vi "Lab Panel V5.29.vi"() -> ()   [LabVIEW 2013] (continued)
            n2896 = Unbundle(w5232) -> ("OUT SERVER ADDRESS"=w5231:string, "FROM ACCOUNT"=w5230:string, "TEST MAIL"=w5229:bool)  [unwired: 4 out]
            n2897 = stacked-sequence {
              tunnel: "TO (string):" -> [_ w5271]
              tunnel: w5232 -> [w5237 w5270]
              tunnel: w5231 -> [w5236 w5269]
              tunnel: w5230 -> [w5235 w5268]
              tunnel: w5229 -> [w5234 _]
              tunnel: w5218 -> [_ w5267]
              tunnel: w5228 -> [_ w5266]
              tunnel: w5227 -> [_ w5265]
              tunnel: w5226 -> [_ w5264]
              tunnel: w5225 -> [_ w5263]
              tunnel: w5224 -> [_ w5262]
              tunnel: w5223 -> [_ w5261]
              tunnel: w5222 -> [_ w5260]
              tunnel: w5221 -> [_ w5259]
              tunnel: w5220 -> [_ w5258]
              tunnel: w5219 -> [_ w5257]
              tunnel: "TO (string):" -> [w5233 _]
              frame #0 {
                # "mail test"
                n2898 = case shown="True" w5234 {
                  tunnel: w5237 -> [_ w5241]
                  tunnel: w5233 -> [_ w5240]
                  tunnel: w5236 -> [_ w5239]
                  tunnel: w5235 -> [_ w5238]
                  frame False {
                  }
                  frame True {
                    n2899 = stacked-sequence {
                      seq-local: [_ _ w5251 _] -> [_ _ _ w5252]
                      tunnel: w5241 -> [w5244 _ _ w5256]
                      tunnel: w5240 -> [_ _ w5249 _]
                      tunnel: w5239 -> [_ _ w5247 _]
                      tunnel: w5238 -> [_ _ w5248 _]
                      frame #0 {
                        n2900 = Bundle(cluster=w5244, "TEST MAIL STATUS"="TEST START") -> (w5242:T7)  [unwired: 6 in]
                        n2901 = local write "MAIL SETTINGS"(w5242) -> ()
                      }
                      frame #1 {
                        n2902 = Wait (ms)(milliseconds to wait=500) -> ()  [unwired: 1 out]
                      }
                      frame #2 {
                        n2903 = call "sub vi - send mail v5.vi"("TO:"=w5249, "subject"="MAIL TEST FROM LAB PANEL", "from"=w5248, "out going server"=w5247, "message"="TEST MESSAGE") -> ("error out"=w5251:errorcluster)  [unwired: 10 in]
                      }
                      frame #3 {
                        n2904 = Bundle(cluster=w5256, "TEST MAIL"=FALSE, "TEST MAIL STATUS"="TEST END", "mail error"=w5252) -> (w5254:T7)  [unwired: 4 in]
                        n2905 = local write "MAIL SETTINGS"(w5254) -> ()
                      }
                    }
                  }
                }
              }
              frame #1 {
                # "mail report"
                n2906 = stacked-sequence {
                  seq-local: [_ w5314 _ _] -> [_ _ _ w5504]
                  seq-local: [_ _ w5417 _] -> [_ _ _ w5494]
                  seq-local: [w5281 _ _ _] -> [_ w5331 _ _]
                  seq-local: [w5280 _ _ _] -> [_ w5330 _ _]
                  seq-local: [w5278 _ _ _] -> [_ w5328 _ _]
                  seq-local: [w5279 _ _ _] -> [_ w5329 _ _]
                  seq-local: [w5277 _ _ _] -> [_ w5327 _ _]
                  seq-local: [w5276 _ _ _] -> [_ w5322 _ _]
                  seq-local: [w5275 _ _ _] -> [_ w5323 _ _]
                  seq-local: [w5274 _ _ _] -> [_ w5324 _ _]
                  seq-local: [w5273 _ _ _] -> [_ w5325 _ _]
                  seq-local: [w5272 _ _ _] -> [_ w5326 _ _]
                  tunnel: w5271 -> [_ _ _ w5505]
                  tunnel: w5270 -> [_ _ _ w5488]
                  tunnel: w5269 -> [_ _ _ w5502]
                  tunnel: w5268 -> [_ _ _ w5501]
                  tunnel: w5267 -> [w5312 _ _ w5496]
                  tunnel: w5266 -> [_ _ w5447 _]
                  tunnel: w5265 -> [_ _ w5444 _]
                  tunnel: w5264 -> [_ _ w5443 _]
                  tunnel: w5263 -> [_ _ w5442 _]
                  tunnel: w5262 -> [_ _ w5441 _]
                  tunnel: w5261 -> [_ _ w5440 _]
                  tunnel: w5260 -> [_ _ w5439 _]
                  tunnel: w5259 -> [_ _ w5438 _]
                  tunnel: w5258 -> [_ _ w5437 _]
                  tunnel: w5257 -> [_ _ w5436 _]
                  frame #0 {
                    n2907 = case shown="False" w5312 {
                      frame False {
                        n2908 = local write "mail control"("") -> ()
                      }
                      frame True {
                      }
                    }
                    n2909 = local read "SET LAB01-1"() -> (w5311:T5)
                    n2910 = local read "SET LAB01-2"() -> (w5310:T5)
                    n2911 = local read "SET LAB02-1"() -> (w5309:T5)
                    n2912 = local read "SET LAB02-2"() -> (w5308:T5)
                    n2913 = local read "SET LAB03-1"() -> (w5307:T5)
                    n2914 = local read "SET LAB04-1"() -> (w5305:T5)
                    n2915 = local read "SET LAB05-1"() -> (w5303:T5)
                    n2916 = local read "SET LAB03-2"() -> (w5306:T5)
                    n2917 = local read "SET LAB04-2"() -> (w5304:T5)
                    n2918 = local read "SET LAB05-2"() -> (w5302:T5)
                    n2919 = Unbundle(w5307) -> ("DESCRIPTION"=w5287:string)  [unwired: 4 out]
                    n2920 = Unbundle(w5306) -> ("DESCRIPTION"=w5286:string)  [unwired: 4 out]
                    n2921 = Unbundle(w5305) -> ("DESCRIPTION"=w5285:string)  [unwired: 4 out]
                    n2922 = Unbundle(w5302) -> ("DESCRIPTION"=w5282:string)  [unwired: 4 out]
                    n2923 = Unbundle(w5308) -> ("DESCRIPTION"=w5288:string)  [unwired: 4 out]
                    n2924 = Unbundle(w5304) -> ("DESCRIPTION"=w5284:string)  [unwired: 4 out]
                    n2925 = Unbundle(w5311) -> ("DESCRIPTION"=w5300:string)  [unwired: 4 out]
                    n2926 = Unbundle(w5309) -> ("DESCRIPTION"=w5289:string)  [unwired: 4 out]
                    n2927 = Unbundle(w5303) -> ("DESCRIPTION"=w5283:string)  [unwired: 4 out]
                    n2928 = Unbundle(w5310) -> ("DESCRIPTION"=w5290:string)  [unwired: 4 out]
                    n2929 = Concatenate Strings("[LAB05-2/", w5282) -> (w5272:string)
                    n2930 = Concatenate Strings("[LAB05-1/", w5283) -> (w5273:string)
                    n2931 = Concatenate Strings("[LAB04-2/", w5284) -> (w5274:string)
                    n2932 = Concatenate Strings("[LAB03-2/", w5286) -> (w5276:string)
                    n2933 = Concatenate Strings("[LAB04-1/", w5285) -> (w5275:string)
                    n2934 = Concatenate Strings("[LAB03-1/", w5287) -> (w5277:string)
                    n2935 = Concatenate Strings("[LAB01-2/", w5290) -> (w5280:string)
                    n2936 = Concatenate Strings("[LAB02-2/", w5288) -> (w5278:string)
                    n2937 = Concatenate Strings("[LAB01-1/", w5300) -> (w5281:string)
                    n2938 = Concatenate Strings("[LAB02-1/", w5289) -> (w5279:string)
                  }
                  frame #1 {
                    w5335 = "/"
                    w5336 = 2.0
                    n2939 = local read "DISP LAB01-2"() -> (w5415:T4)
                    n2940 = local read "DISP LAB01-1"() -> (w5416:T4)
                    n2941 = local read "DISP LAB02-1"() -> (w5414:T4)
                    n2942 = local read "DISP LAB03-2"() -> (w5411:T4)
                    n2943 = local read "DISP LAB02-2"() -> (w5413:T4)
                    n2944 = local read "DISP LAB03-1"() -> (w5412:T4)
                    n2945 = local read "DISP LAB04-2"() -> (w5409:T4)
                    n2946 = local read "DISP LAB04-1"() -> (w5410:T4)
                    n2947 = local read "DISP LAB05-1"() -> (w5408:T4)
                    n2948 = local read "DISP LAB05-2"() -> (w5407:T4)
                    n2949 = Unbundle(w5415) -> ("CYCLE"=w5399:dbl, "MINS"=w5398:dbl, "STATUS"=w5395:string)
                    n2950 = Unbundle(w5416) -> ("CYCLE"=w5404:dbl, "MINS"=w5403:dbl, "STATUS"=w5400:string)
                    n2951 = Unbundle(w5414) -> ("CYCLE"=w5392:dbl, "MINS"=w5391:dbl, "STATUS"=w5390:string)
                    n2952 = Unbundle(w5411) -> ("CYCLE"=w5379:dbl, "MINS"=w5378:dbl, "STATUS"=w5375:string)
                    n2953 = Unbundle(w5412) -> ("CYCLE"=w5384:dbl, "MINS"=w5383:dbl, "STATUS"=w5380:string)
                    n2954 = Unbundle(w5413) -> ("CYCLE"=w5389:dbl, "MINS"=w5388:dbl, "STATUS"=w5385:string)
                    n2955 = Unbundle(w5410) -> ("CYCLE"=w5374:dbl, "MINS"=w5373:dbl, "STATUS"=w5370:string)
                    n2956 = Unbundle(w5409) -> ("CYCLE"=w5369:dbl, "MINS"=w5368:dbl, "STATUS"=w5365:string)
                    n2957 = Unbundle(w5408) -> ("CYCLE"=w5364:dbl, "MINS"=w5363:dbl, "STATUS"=w5360:string)
                    n2958 = Unbundle(w5407) -> ("CYCLE"=w5406:dbl, "MINS"=w5405:dbl, "STATUS"=w5357:string)
                    n2959 = Number To Decimal String(number=w5392) -> (decimal integer string=w5394:string)  [unwired: 1 in]
                    n2960 = Number To Decimal String(number=w5389) -> (decimal integer string=w5387:string)  [unwired: 1 in]
                    n2961 = Number To Decimal String(number=w5384) -> (decimal integer string=w5382:string)  [unwired: 1 in]
                    n2962 = Number To Decimal String(number=w5399) -> (decimal integer string=w5397:string)  [unwired: 1 in]
                    n2963 = Number To Decimal String(number=w5379) -> (decimal integer string=w5377:string)  [unwired: 1 in]
                    n2964 = Number To Decimal String(number=w5404) -> (decimal integer string=w5402:string)  [unwired: 1 in]
                    n2965 = Number To Decimal String(number=w5406) -> (decimal integer string=w5359:string)  [unwired: 1 in]
                    n2966 = Number To Decimal String(number=w5374) -> (decimal integer string=w5372:string)  [unwired: 1 in]
                    n2967 = Number To Decimal String(number=w5369) -> (decimal integer string=w5367:string)  [unwired: 1 in]
                    n2968 = Number To Decimal String(number=w5364) -> (decimal integer string=w5362:string)  [unwired: 1 in]
                    n2969 = Number To Fractional String(number=w5391, precision (6)=w5336) -> (F-format string=w5393:string)  [unwired: 2 in]
                    n2970 = Number To Fractional String(number=w5378, precision (6)=w5336) -> (F-format string=w5376:string)  [unwired: 2 in]
                    n2971 = Number To Fractional String(number=w5388, precision (6)=w5336) -> (F-format string=w5386:string)  [unwired: 2 in]
                    n2972 = Number To Fractional String(number=w5383, precision (6)=w5336) -> (F-format string=w5381:string)  [unwired: 2 in]
                    n2973 = Number To Fractional String(number=w5368, precision (6)=w5336) -> (F-format string=w5366:string)  [unwired: 2 in]
                    n2974 = Number To Fractional String(number=w5373, precision (6)=w5336) -> (F-format string=w5371:string)  [unwired: 2 in]
                    n2975 = Number To Fractional String(number=w5398, precision (6)=w5336) -> (F-format string=w5396:string)  [unwired: 2 in]
                    n2976 = Number To Fractional String(number=w5363, precision (6)=w5336) -> (F-format string=w5361:string)  [unwired: 2 in]
                    n2977 = Number To Fractional String(number=w5403, precision (6)=w5336) -> (F-format string=w5401:string)  [unwired: 2 in]
                    n2978 = Number To Fractional String(number=w5405, precision (6)=w5336) -> (F-format string=w5358:string)  [unwired: 2 in]
                    n2979 = Concatenate Strings(w5335, w5377, w5335, w5376, w5335, w5375) -> (w5351:string)
                    n2980 = Concatenate Strings(w5335, w5372, w5335, w5371, w5335, w5370) -> (w5350:string)
                    n2981 = Concatenate Strings(w5335, w5367, w5335, w5366, w5335, w5365) -> (w5349:string)
                    n2982 = Concatenate Strings(w5335, w5362, w5335, w5361, w5335, w5360) -> (w5348:string)
                    n2983 = Concatenate Strings(w5335, w5359, w5335, w5358, w5335, w5357) -> (w5347:string)
                    n2984 = Concatenate Strings(w5335, w5402, w5335, w5401, w5335, w5400) -> (w5356:string)
                    n2985 = Concatenate Strings(w5335, w5382, w5335, w5381, w5335, w5380) -> (w5352:string)
                    n2986 = Concatenate Strings(w5335, w5397, w5335, w5396, w5335, w5395) -> (w5355:string)
                    n2987 = Concatenate Strings(w5335, w5394, w5335, w5393, w5335, w5390) -> (w5354:string)
                    n2988 = Concatenate Strings(w5335, w5387, w5335, w5386, w5335, w5385) -> (w5353:string)
                    n2989 = Concatenate Strings("]", "\r") -> (w5332:string)
                    n2990 = Concatenate Strings(w5327, w5352, w5332) -> (w5342:string)
                    n2991 = Concatenate Strings(w5329, w5354, w5332) -> (w5344:string)
                    n2992 = Concatenate Strings(w5328, w5353, w5332) -> (w5343:string)
                    n2993 = Concatenate Strings(w5324, w5349, w5332) -> (w5339:string)
                    n2994 = Concatenate Strings(w5325, w5348, w5332) -> (w5340:string)
                    n2995 = Concatenate Strings(w5323, w5350, w5332) -> (w5338:string)
                    n2996 = Concatenate Strings(w5322, w5351, w5332) -> (w5337:string)
                    n2997 = Concatenate Strings(w5326, w5347, w5332) -> (w5341:string)
                    n2998 = Concatenate Strings(w5330, w5355, w5332) -> (w5345:string)
                    n2999 = Concatenate Strings(w5331, w5356, w5332) -> (w5346:string)
                    n3000 = Concatenate Strings(w5346, w5345, w5344, w5343, w5342, w5337, w5338, w5339, w5340, w5341) -> (w5315:string)
                    n3001 = Concatenate Strings("[PANEL/", "DESC/", "CYCLES/", "MINS/", "STATUS]", "\r", w5315) -> (w5314:string)
                    "MAIL REPORT" <- w5314
                    n3002 = global write "Global display 3.vi" "log all"(w5314) -> ()
                  }
                  frame #2 {
                    w5445 = "END"
                    n3003 = local read "mail control"() -> (w5446:string)
                    n3004 = case shown="False" w5441 {
                      tunnel: w5446 -> [w5470 _]
                      tunnel: w5445 -> [w5469 _]
                      tunnel: [w5468 FALSE] -> w5431
                      frame False {
                        n3005 = Equal?(x=w5470, y=w5469) -> (x = y?=w5468:bool)
                      }
                      frame True {
                      }
                    }
                    n3006 = case shown="False" w5447 {
                      tunnel: w5446 -> [w5486 _]
                      tunnel: w5445 -> [w5485 _]
                      tunnel: [w5484 FALSE] -> w5435
                      frame False {
                        n3007 = Equal?(x=w5486, y=w5485) -> (x = y?=w5484:bool)
                      }
                      frame True {
                      }
                    }
                    n3008 = case shown="False" w5444 {
                      tunnel: w5446 -> [w5482 _]
                      tunnel: w5445 -> [w5481 _]
                      tunnel: [w5480 FALSE] -> w5434
                      frame False {
                        n3009 = Equal?(x=w5482, y=w5481) -> (x = y?=w5480:bool)
                      }
                      frame True {
                      }
                    }
                    n3010 = case shown="False" w5442 {
                      tunnel: w5446 -> [w5474 _]
                      tunnel: w5445 -> [w5473 _]
                      tunnel: [w5472 FALSE] -> w5432
                      frame False {
                        n3011 = Equal?(x=w5474, y=w5473) -> (x = y?=w5472:bool)
                      }
                      frame True {
                      }
                    }
                    n3012 = case shown="False" w5443 {
                      tunnel: w5446 -> [w5478 _]
                      tunnel: w5445 -> [w5477 _]
                      tunnel: [w5476 FALSE] -> w5433
                      frame False {
                        n3013 = Equal?(x=w5478, y=w5477) -> (x = y?=w5476:bool)
                      }
                      frame True {
                      }
                    }
                    n3014 = Or(x=w5433, y=w5432) -> (x .or. y?=w5424:bool)
                    n3015 = Or(x=w5435, y=w5434) -> (x .or. y?=w5425:bool)
                    n3016 = Or(x=w5425, y=w5424) -> (x .or. y?=w5420:bool)
                    n3017 = case shown="False" w5437 {
                      tunnel: w5446 -> [w5454 _]
                      tunnel: w5445 -> [w5453 _]
                      tunnel: [w5452 FALSE] -> w5426
                      frame False {
                        n3018 = Equal?(x=w5454, y=w5453) -> (x = y?=w5452:bool)
                      }
                      frame True {
                      }
                    }
                    n3019 = case shown="False" w5436 {
                      tunnel: w5446 -> [w5450 _]
                      tunnel: w5445 -> [w5449 _]
                      tunnel: [w5448 FALSE] -> w5430
                      frame False {
                        n3020 = Equal?(x=w5450, y=w5449) -> (x = y?=w5448:bool)
                      }
                      frame True {
                      }
                    }
                    n3021 = case shown="False" w5438 {
                      tunnel: w5446 -> [w5458 _]
                      tunnel: w5445 -> [w5457 _]
                      tunnel: [w5456 FALSE] -> w5427
                      frame False {
                        n3022 = Equal?(x=w5458, y=w5457) -> (x = y?=w5456:bool)
                      }
                      frame True {
                      }
                    }
                    n3023 = case shown="False" w5440 {
                      tunnel: w5446 -> [w5466 _]
                      tunnel: w5445 -> [w5465 _]
                      tunnel: [w5464 FALSE] -> w5429
                      frame False {
                        n3024 = Equal?(x=w5466, y=w5465) -> (x = y?=w5464:bool)
                      }
                      frame True {
                      }
                    }
                    n3025 = case shown="False" w5439 {
                      tunnel: w5446 -> [w5462 _]
                      tunnel: w5445 -> [w5461 _]
                      tunnel: [w5460 FALSE] -> w5428
                      frame False {
                        n3026 = Equal?(x=w5462, y=w5461) -> (x = y?=w5460:bool)
                      }
                      frame True {
                      }
                    }
                    n3027 = Or(x=w5429, y=w5428) -> (x .or. y?=w5423:bool)
                    n3028 = Or(x=w5427, y=w5426) -> (x .or. y?=w5422:bool)
                    n3029 = Or(x=w5430, y=w5431) -> (x .or. y?=w5418:bool)
                    n3030 = Or(x=w5423, y=w5422) -> (x .or. y?=w5421:bool)
                    n3031 = Or(x=w5420, y=w5421) -> (x .or. y?=w5419:bool)
                    n3032 = Or(x=w5419, y=w5418) -> (x .or. y?=w5417:bool)
                  }
                  frame #3 {
                    n3033 = local read "on loops"() -> (w5500:dbl)
                    n3034 = local read "jig cycle"() -> (w5497:dbl)
                    n3035 = local read "Send Mail Now"() -> (w5491:bool)
                    n3036 = Add(x=w5500, y=5.0) -> (x+y=w5498:dbl)
                    n3037 = Equal?(x=w5497, y=w5498) -> (x = y?=w5492:bool)
                    n3038 = And(x=w5492, y=w5491) -> (x .and. y?=w5490:bool)
                    n3039 = And(x=w5496, y=w5492) -> (x .and. y?=w5495:bool)
                    n3040 = And(x=w5495, y=w5494) -> (x .and. y?=w5493:bool)
                    n3041 = Or(x=w5493, y=w5490) -> (x .or. y?=w5489:bool)
                    n3042 = case shown="True" w5489 {
                      tunnel: w5505 -> [_ w5511]
                      tunnel: w5504 -> [_ w5510]
                      tunnel: "Lab Panel Test Status" -> [_ w5509]
                      tunnel: w5502 -> [_ w5508]
                      tunnel: w5501 -> [_ w5507]
                      tunnel: w5488 -> [_ w5506]
                      frame False {
                      }
                      frame True {
                        n3043 = stacked-sequence {
                          tunnel: w5511 -> [w5520 _]
                          tunnel: w5510 -> [w5519 _]
                          tunnel: w5509 -> [w5518 _]
                          tunnel: w5508 -> [w5517 _]
                          tunnel: w5507 -> [w5516 _]
                          tunnel: w5506 -> [w5515 _]
                          frame #0 {
                            n3044 = call "sub vi - send mail v5.vi"("TO:"=w5520, "subject"=w5518, "Info"="Test station status report", "from"=w5516, "out going server"=w5517, "message"=w5519) -> ("error out"=w5514:errorcluster)  [unwired: 9 in]
                            n3045 = Bundle(cluster=w5515, "mail error"=w5514) -> (w5513:T7)  [unwired: 6 in]
                            n3046 = local write "MAIL SETTINGS"(w5513) -> ()
                          }
                          frame #1 {
                            n3047 = local write "mail control"("") -> ()
                            n3048 = local write "Send Mail Now"(FALSE) -> ()
                          }
                        }
                      }
                    }
                  }
                }
              }
            }
          }
          frame #20 {
            # "save jig cycle values once all run switches are off"
            n3049 = stacked-sequence {
              tunnel: w5532 -> [_ w5561]
              tunnel: w5531 -> [_ w5560]
              tunnel: w5530 -> [_ w5559]
              tunnel: w5529 -> [_ w5558]
              tunnel: w5528 -> [_ w5557]
              tunnel: w5527 -> [_ w5556]
              tunnel: w5526 -> [_ w5555]
              tunnel: w5525 -> [_ w5554]
              tunnel: w5524 -> [_ w5553]
              tunnel: w5523 -> [_ w5552]
              frame #0 {
              }
              frame #1 {
                n3050 = Not(x=w5552) -> (.not. x?=w5535:bool)
                n3051 = Not(x=w5560) -> (.not. x?=w5550:bool)
                n3052 = Not(x=w5557) -> (.not. x?=w5545:bool)
                n3053 = Not(x=w5555) -> (.not. x?=w5541:bool)
                n3054 = Not(x=w5553) -> (.not. x?=w5537:bool)
                n3055 = Not(x=w5561) -> (.not. x?=w5551:bool)
                n3056 = Not(x=w5559) -> (.not. x?=w5549:bool)
                n3057 = Not(x=w5556) -> (.not. x?=w5543:bool)
                n3058 = Not(x=w5558) -> (.not. x?=w5547:bool)
                n3059 = Not(x=w5554) -> (.not. x?=w5539:bool)
                n3060 = local read "Save JC"() -> (w5563:bool)
                n3061 = And(x=w5551, y=w5550) -> (x .and. y?=w5548:bool)
                n3062 = And(x=w5548, y=w5549) -> (x .and. y?=w5546:bool)
                n3063 = And(x=w5546, y=w5547) -> (x .and. y?=w5544:bool)
                n3064 = And(x=w5544, y=w5545) -> (x .and. y?=w5542:bool)
                n3065 = And(x=w5542, y=w5543) -> (x .and. y?=w5540:bool)
                n3066 = And(x=w5540, y=w5541) -> (x .and. y?=w5538:bool)
                n3067 = And(x=w5538, y=w5539) -> (x .and. y?=w5536:bool)
                n3068 = And(x=w5536, y=w5537) -> (x .and. y?=w5534:bool)
                n3069 = And(x=w5534, y=w5535) -> (x .and. y?=w5533:bool)
                n3070 = And(x=w5533, y=w5563) -> (x .and. y?=w5562:bool)
                n3071 = case shown="True" w5562 {
                  tunnel: w5533 -> [w5564 _]
                  frame False {
                    n3072 = case shown="False" w5564 {
                      frame False {
                        n3073 = local write "Save JC"(TRUE) -> ()
                      }
                      frame True {
                      }
                    }
                  }
                  frame True {
                    n3074 = stacked-sequence {
                      frame #0 {
                        n3075 = String To Path(string="c:\\crabtree\\Jig Cycles\\") -> (path=w5576:path)
                        n3076 = Build Path(base path=w5576, name or relative path="jigcycles.bin") -> (appended path=w5574:path)
                        n3077 = Create Folder(path (use dialog)=w5576) -> (error out=w5578:errorcluster)  [unwired: 2 in, 2 out]
                        n3078 = local read "JIG RELAY CYCLES"() -> (w5568:T8)
                        n3079 = call <vilib>:"Clear Errors.vi"("error in (no error)"=w5578) -> ()  [unwired: 6 in, 1 out]
                        n3080 = local write "Save JC"(FALSE) -> ()
                        n3081 = Open/Create/Replace File(file path (use dialog)=w5574, operation (0:open)=T17."replace or create") -> (refnum out=w5572:refnum<file>, error out=w5573:errorcluster)  [unwired: 4 in, 1 out]
                        n3082 = Write to Binary File(file (use dialog)=w5572, data=w5568, error in=w5573) -> (refnum out=w5571:refnum<file>, error out=w5570:errorcluster)  [unwired: 3 in, 1 out]
                        n3083 = Close File(refnum=w5571, error in=w5570) -> (error out=w5569:errorcluster)  [unwired: 1 out]
                        n3084 = local write "data file error"(w5569) -> ()
                      }
                      frame #1 {
                        n3085 = local read "JIG RELAY CYCLES"() -> (w5601:T8)
                        n3086 = Unbundle By Name(w5601) -> ("LAB01-1"=w5596:dbl, "LAB01-2"=w5595:dbl, "LAB02-1"=w5593:dbl, "LAB02-2"=w5592:dbl, "LAB03-1"=w5590:dbl, "LAB03-2"=w5587:dbl, "LAB04-1"=w5586:dbl, "LAB04-2"=w5584:dbl, "LAB05-1"=w5582:dbl, "LAB05-2"=w5580:dbl)
                        n3087 = stacked-sequence {
                          tunnel: w5596 -> [w5604 _ _ _ _ _ _ _ _ _]
                          tunnel: 1000000 -> [w5607 w5617 w5627 w5637 w5647 w5657 w5667 w5677 w5687 w5697]
                          tunnel: [w5605 _ _ _ _ _ _ _ _ _] -> w5599
                          tunnel: "TEST STATION HAS REACHED 1 MILLION CYCLES, REPLACE  CONTROL RELAYS" -> [w5603 w5615 w5625 w5635 w5645 w5655 w5665 w5675 w5685 w5695]
                          tunnel: [_ w5614 _ _ _ _ _ _ _ _] -> w5597
                          tunnel: w5595 -> [_ w5613 _ _ _ _ _ _ _ _]
                          tunnel: [_ _ w5624 _ _ _ _ _ _ _] -> w5594
                          tunnel: w5593 -> [_ _ w5623 _ _ _ _ _ _ _]
                          tunnel: w5592 -> [_ _ _ w5634 _ _ _ _ _ _]
                          tunnel: [_ _ _ w5633 _ _ _ _ _ _] -> w5591
                          tunnel: w5590 -> [_ _ _ _ w5644 _ _ _ _ _]
                          tunnel: [_ _ _ _ w5643 _ _ _ _ _] -> w5589
                          tunnel: [_ _ _ _ _ w5654 _ _ _ _] -> w5588
                          tunnel: w5587 -> [_ _ _ _ _ w5653 _ _ _ _]
                          tunnel: w5586 -> [_ _ _ _ _ _ w5664 _ _ _]
                          tunnel: [_ _ _ _ _ _ w5663 _ _ _] -> w5585
                          tunnel: w5584 -> [_ _ _ _ _ _ _ w5674 _ _]
                          tunnel: [_ _ _ _ _ _ _ w5673 _ _] -> w5583
                          tunnel: w5582 -> [_ _ _ _ _ _ _ _ w5684 _]
                          tunnel: [_ _ _ _ _ _ _ _ w5683 _] -> w5581
                          tunnel: w5580 -> [_ _ _ _ _ _ _ _ _ w5694]
                          tunnel: [_ _ _ _ _ _ _ _ _ w5693] -> w5579
                          frame #0 {
                            n3088 = Greater?(x=w5604, y=w5607) -> (0:w5606:bool)
                            n3089 = case shown="True" w5606 {
                              tunnel: [w5608 0] -> w5605
                              tunnel: w5604 -> [w5608 _]
                              tunnel: w5603 -> [_ w5609]
                              frame False {
                              }
                              frame True {
                                n3090 = Concatenate Strings("LA01-1 ", w5609) -> (w5612:string)
                                n3091 = One Button Dialog(message=w5612) -> ()  [unwired: 1 in, 1 out]
                              }
                            }
                          }
                          frame #1 {
                            n3092 = Greater?(x=w5613, y=w5617) -> (0:w5616:bool)
                            n3093 = case shown="True" w5616 {
                              tunnel: [w5618 0] -> w5614
                              tunnel: w5613 -> [w5618 _]
                              tunnel: w5615 -> [_ w5619]
                              frame False {
                              }
                              frame True {
                                n3094 = Concatenate Strings("LA01-2 ", w5619) -> (w5622:string)
                                n3095 = One Button Dialog(message=w5622) -> ()  [unwired: 1 in, 1 out]
                              }
                            }
                          }
                          frame #2 {
                            n3096 = Greater?(x=w5623, y=w5627) -> (0:w5626:bool)
                            n3097 = case shown="True" w5626 {
                              tunnel: [w5628 0] -> w5624
                              tunnel: w5623 -> [w5628 _]
                              tunnel: w5625 -> [_ w5629]
                              frame False {
                              }
                              frame True {
                                n3098 = Concatenate Strings("LA02-1 ", w5629) -> (w5632:string)
                                n3099 = One Button Dialog(message=w5632) -> ()  [unwired: 1 in, 1 out]
                              }
                            }
                          }
                          frame #3 {
                            n3100 = Greater?(x=w5634, y=w5637) -> (0:w5636:bool)
                            n3101 = case shown="True" w5636 {
                              tunnel: [w5638 0] -> w5633
                              tunnel: w5634 -> [w5638 _]
                              tunnel: w5635 -> [_ w5639]
                              frame False {
                              }
                              frame True {
                                n3102 = Concatenate Strings("LA02-2 ", w5639) -> (w5642:string)
                                n3103 = One Button Dialog(message=w5642) -> ()  [unwired: 1 in, 1 out]
                              }
                            }
                          }
                          frame #4 {
                            n3104 = Greater?(x=w5644, y=w5647) -> (0:w5646:bool)
                            n3105 = case shown="True" w5646 {
                              tunnel: [w5648 0] -> w5643
                              tunnel: w5644 -> [w5648 _]
                              tunnel: w5645 -> [_ w5649]
                              frame False {
                              }
                              frame True {
                                n3106 = Concatenate Strings("LA03-1 ", w5649) -> (w5652:string)
                                n3107 = One Button Dialog(message=w5652) -> ()  [unwired: 1 in, 1 out]
                              }
                            }
                          }
                          frame #5 {
                            n3108 = Greater?(x=w5653, y=w5657) -> (0:w5656:bool)
                            n3109 = case shown="True" w5656 {
                              tunnel: [w5658 0] -> w5654
                              tunnel: w5653 -> [w5658 _]
                              tunnel: w5655 -> [_ w5659]
                              frame False {
                              }
                              frame True {
                                n3110 = Concatenate Strings("LA03-2 ", w5659) -> (w5662:string)
                                n3111 = One Button Dialog(message=w5662) -> ()  [unwired: 1 in, 1 out]
                              }
                            }
                          }
                          frame #6 {
                            n3112 = Greater?(x=w5664, y=w5667) -> (0:w5666:bool)
                            n3113 = case shown="True" w5666 {
                              tunnel: [w5668 0] -> w5663
                              tunnel: w5664 -> [w5668 _]
                              tunnel: w5665 -> [_ w5669]
                              frame False {
                              }
                              frame True {
                                n3114 = Concatenate Strings("LA04-1 ", w5669) -> (w5672:string)
                                n3115 = One Button Dialog(message=w5672) -> ()  [unwired: 1 in, 1 out]
                              }
                            }
                          }
                          frame #7 {
                            n3116 = Greater?(x=w5674, y=w5677) -> (0:w5676:bool)
                            n3117 = case shown="True" w5676 {
                              tunnel: [w5678 0] -> w5673
                              tunnel: w5674 -> [w5678 _]
                              tunnel: w5675 -> [_ w5679]
                              frame False {
                              }
                              frame True {
                                n3118 = Concatenate Strings("LA04-2 ", w5679) -> (w5682:string)
                                n3119 = One Button Dialog(message=w5682) -> ()  [unwired: 1 in, 1 out]
                              }
                            }
                          }
                          frame #8 {
                            n3120 = Greater?(x=w5684, y=w5687) -> (0:w5686:bool)
                            n3121 = case shown="True" w5686 {
                              tunnel: [w5688 0] -> w5683
                              tunnel: w5684 -> [w5688 _]
                              tunnel: w5685 -> [_ w5689]
                              frame False {
                              }
                              frame True {
                                n3122 = Concatenate Strings("LA05-1 ", w5689) -> (w5692:string)
                                n3123 = One Button Dialog(message=w5692) -> ()  [unwired: 1 in, 1 out]
                              }
                            }
                          }
                          frame #9 {
                            n3124 = Greater?(x=w5694, y=w5697) -> (0:w5696:bool)
                            n3125 = case shown="True" w5696 {
                              tunnel: [w5698 0] -> w5693
                              tunnel: w5694 -> [w5698 _]
                              tunnel: w5695 -> [_ w5699]
                              frame False {
                              }
                              frame True {
                                n3126 = Concatenate Strings("LA05-2 ", w5699) -> (w5702:string)
                                n3127 = One Button Dialog(message=w5702) -> ()  [unwired: 1 in, 1 out]
                              }
                            }
                          }
                        }
                        n3128 = Bundle By Name(cluster=w5601, "LAB01-1"=w5599, "LAB01-2"=w5597, "LAB02-1"=w5594, "LAB02-2"=w5591, "LAB03-1"=w5589, "LAB03-2"=w5588, "LAB04-1"=w5585, "LAB04-2"=w5583, "LAB05-1"=w5581, "LAB05-2"=w5579) -> (w5600:T8)
                        n3129 = local write "JIG RELAY CYCLES"(w5600) -> ()
                      }
                    }
                  }
                }
              }
            }
          }
          frame #21 {
            # "get temperature values"
            n3130 = local read "Simulate"() -> (w5715:bool)
            n3131 = local read "Temp Test Cal"() -> (w5712:dbl)
            n3132 = stacked-sequence {
              seq-local: [_ w5722 _] -> [_ _ w5767]
              tunnel: w5715 -> [_ _ w5780]
              tunnel: T14 {"1  (A) cal"=1.0, "1 (V) cal"=1.0, "1 (PF) cal"=1.0, "1 (TL) cal"=1.0, "1 (TN) cal"=1.0, "2 (A) cal"=1.0, "2 (V) cal"=1.0, "2 (PF) cal"=1.0, "2 (TL) cal"=1.0, "2 (TN) cal"=1.0} ("CAL LAB01") -> [_ _ w5779]
              tunnel: w5713 -> [_ _ w5778]
              tunnel: w5712 -> [_ _ w5777]
              tunnel: w5711 -> [_ _ w5776]
              tunnel: w5710 -> [_ _ w5775]
              tunnel: w5709 -> [_ _ w5774]
              tunnel: w5708 -> [_ _ w5773]
              tunnel: w5707 -> [_ _ w5772]
              tunnel: w5706 -> [_ _ w5771]
              tunnel: w5705 -> [_ _ w5770]
              tunnel: w5704 -> [_ _ w5769]
              tunnel: w5703 -> [_ _ w5768]
              frame #0 {
                n3133 = case shown="True" "Open Com Port" {
                  frame False {
                  }
                  frame True {
                    n3134 = local read "Select COM port"() -> (w5720:refnum<visa-resource-name>)
                    n3135 = call "sub vi-open serial port v1.vi"("Select COM port"=w5720) -> ("status"=w5719:bool, "LOOPS"=w5718:i32, "VISA Com out"=w5717:refnum<visa-resource-name>)  [unwired: 12 in]
                    n3136 = local write "Com setup loops"(w5718) -> ()
                    n3137 = local write "Com Port Status"(w5719) -> ()
                    n3138 = local write "VISA Com out"(w5717) -> ()
                    n3139 = global write "Global 1.vi" "COM port"(w5717) -> ()
                  }
                }
              }
              frame #1 {
                # "only get temperature from initial valid temperature circuits"
                n3140 = local read "VISA Com out"() -> (w5730:refnum<visa-resource-name>)
                n3141 = global write "Global 1.vi" "COM port"(w5730) -> ()
                n3142 = local read "Temp read loop"() -> (w5727:dbl)
                n3143 = global write "Global 1.vi" "tmp dly lps"("Temp Delay Lps") -> ()
                n3144 = global write "Global 1.vi" "dly value"("Temp Value") -> ()
                n3145 = local read "jig cycle"() -> (w5731:dbl)
                n3146 = local read "on loops"() -> (w5733:dbl)
                n3147 = Equal?(x=w5727, y=1) -> (x = y?=w5724:bool)
                n3148 = Add(x=w5733, y=6) -> (x+y=w5734:dbl)
                n3149 = Equal?(x=w5731, y=w5734) -> (x = y?=w5725:bool)
                n3150 = And(x=w5725, y=w5724) -> (x .and. y?=w5723:bool)
                n3151 = Or(x=w5723, y="Read Temp") -> (x .or. y?=w5722:bool)
                n3152 = case shown="True" w5722 {
                  frame False {
                  }
                  frame True {
                    n3153 = local read "Simulate"() -> (w5736:bool)
                    n3154 = local write "TEMP"(TRUE) -> ()
                    n3155 = local write "Read Temp"(FALSE) -> ()
                    n3156 = stacked-sequence {
                      tunnel: 1.0 -> [_ _ _ _ w5766]
                      tunnel: w5736 -> [_ _ _ _ w5765]
                      frame #0 {
                        # "only switch relay on to reset temp circuits if busy testing"
                        n3157 = disable-structure shown="Disabled" {
                          frame Disabled {
                            n3158 = local read "Any Test Running"() -> ()  [unwired: 1 out]
                          }
                          frame Enabled {
                          }
                        }
                        n3159 = local read "USB OUT 0"() -> (w5740:bool[])
                        n3160 = local read "USB OUT 2"() -> (w5742:bool[])
                        n3161 = local read "USB OUT 1"() -> (w5741:bool[])
                        n3162 = Insert Into Array(array=w5742, index=7, new element=TRUE) -> (w5743:bool[])
                        n3163 = call "sub vi - Drive Relays All v6.vi"("Array #2"=w5743, "Array #1"=w5741, "Array #0"=w5740) -> ()  [unwired: 8 in, 1 out]
                      }
                      frame #1 {
                        # "time delay"
                        n3164 = Wait (ms)(milliseconds to wait=500) -> ()  [unwired: 1 out]
                      }
                      frame #2 {
                        # "switch relay off"
                        n3165 = local read "USB OUT 0"() -> (w5746:bool[])
                        n3166 = local read "USB OUT 2"() -> (w5748:bool[])
                        n3167 = local read "USB OUT 1"() -> (w5747:bool[])
                        n3168 = Insert Into Array(array=w5748, index=7, new element=FALSE) -> (w5749:bool[])
                        n3169 = call "sub vi - Drive Relays All v6.vi"("Array #2"=w5749, "Array #1"=w5747, "Array #0"=w5746) -> ()  [unwired: 8 in, 1 out]
                      }
                      frame #3 {
                        # "time delay"
                        n3170 = Wait (ms)(milliseconds to wait=300) -> ()  [unwired: 1 out]
                      }
                      frame #4 {
                        # "read all valid temp circuits"
                        n3171 = local read "LAB01-TP"() -> (w5758:bool)
                        n3172 = local read "LAB03-TP"() -> (w5756:bool)
                        n3173 = local read "LAB02-TP"() -> (w5757:bool)
                        n3174 = local read "LAB04-TP"() -> (w5755:bool)
                        n3175 = local read "LAB05-TP"() -> (w5759:bool)
                        n3176 = call "sub vi - GET ALL TEMP v7.vi"("LA01-EN"=w5758, "simulate"=w5765, "LA02-EN"=w5757, "LA03-EN"=w5756, "LA04-EN"=w5755, "LA05-EN"=w5759, "Gen Cal Value"=w5766) -> ("LOOP TIME"=→"Read Time":dbl, "LA01 TEMP"=w5764:T25, "LA02 TEMP"=w5763:T25, "LA03 TEMP"=w5762:T25, "LA04 TEMP"=w5761:T25, "error"=→"Error Temp":bool, "LA05 TEMP"=w5760:T25)  [unwired: 1 in, 1 out]
                        n3177 = local write "LAB01 TEMP"(w5764) -> ()
                        n3178 = local write "LAB02 TEMP"(w5763) -> ()
                        n3179 = local write "LAB03 TEMP"(w5762) -> ()
                        n3180 = local write "LAB04 TEMP"(w5761) -> ()
                        n3181 = local write "LAB05 TEMP"(w5760) -> ()
                      }
                    }
                  }
                }
              }
              frame #2 {
                n3182 = case shown="True" w5767 {
                  tunnel: w5780 -> [_ w5793]
                  tunnel: w5779 -> [_ w5792]
                  tunnel: w5778 -> [_ w5791]
                  tunnel: w5777 -> [_ w5790]
                  tunnel: w5776 -> [_ w5789]
                  tunnel: w5775 -> [_ w5788]
                  tunnel: w5774 -> [_ w5787]
                  tunnel: w5773 -> [_ w5786]
                  tunnel: w5772 -> [_ w5785]
                  tunnel: w5771 -> [_ w5784]
                  tunnel: w5770 -> [_ w5783]
                  tunnel: w5769 -> [_ w5782]
                  tunnel: w5768 -> [_ w5781]
                  frame False {
                  }
                  frame True {
                    n3183 = stacked-sequence {
                      tunnel: w5793 -> [_ w5806 w5851 w5896 w5941 w5986 _]
                      tunnel: w5792 -> [_ w5805 w5850 w5895 w5940 w5985 _]
                      tunnel: w5791 -> [_ w5795 _ _ _ _ _]
                      tunnel: w5790 -> [_ w5800 w5849 w5894 w5939 w5984 _]
                      tunnel: w5789 -> [_ w5794 _ _ _ _ _]
                      tunnel: w5788 -> [_ _ w5840 _ _ _ _]
                      tunnel: w5787 -> [_ _ w5839 _ _ _ _]
                      tunnel: w5786 -> [_ _ _ w5885 _ _ _]
                      tunnel: w5785 -> [_ _ _ w5884 _ _ _]
                      tunnel: w5784 -> [_ _ _ _ w5930 _ _]
                      tunnel: w5783 -> [_ _ _ _ w5929 _ _]
                      tunnel: w5782 -> [_ _ _ _ _ w5975 _]
                      tunnel: w5781 -> [_ _ _ _ _ w5974 _]
                      frame #0 {
                      }
                      frame #1 {
                        n3184 = case shown="False" w5806 {
                          tunnel: [w5837 w5838] -> w5822
                          tunnel: w5805 -> [_ w5838]
                          frame False {
                            n3185 = local read "CAL LAB01"() -> (w5837:T14)
                          }
                          frame True {
                          }
                        }
                        n3186 = local read "TEMP LA01"() -> (w5813:T9)
                        n3187 = local read "LAB01 TEMP"() -> (w5812:T12)
                        n3188 = call "sub vi - temperature delay v4.vi"("2-run"=w5794, "1-run"=w5795, "temp values IN"=w5813, "temp signals"=w5812) -> ("T2-N"=w5808:dbl, "T2-L"=w5809:dbl, "T1-N"=w5810:dbl, "T1-L"=w5811:dbl, "temp values OUT"=w5807:T44)  [unwired: 3 in]
                        n3189 = Unbundle By Name(w5822) -> ("1 (TL) cal"=w5817:dbl, "1 (TN) cal"=w5816:dbl, "2 (TL) cal"=w5815:dbl, "2 (TN) cal"=w5814:dbl)  [unwired: 6 out]
                        n3190 = local write "TEMP LA01"(w5807) -> ()
                        n3191 = Multiply(x=w5811, y=w5817) -> (x*y=w5804:dbl)
                        n3192 = Multiply(x=w5810, y=w5816) -> (x*y=w5802:dbl)
                        n3193 = Multiply(x=w5809, y=w5815) -> (x*y=w5799:dbl)
                        n3194 = Multiply(x=w5808, y=w5814) -> (x*y=w5798:dbl)
                        n3195 = case shown="True" w5795 {
                          tunnel: w5804 -> [w5831 w5836]
                          tunnel: w5800 -> [_ w5834]
                          tunnel: [w5831 w5835] -> w5803
                          tunnel: w5802 -> [w5830 w5833]
                          tunnel: [w5830 w5832] -> w5801
                          frame False {
                          }
                          frame True {
                            n3196 = Multiply(x=w5834, y=w5833) -> (x*y=w5832:dbl)
                            n3197 = Multiply(x=w5834, y=w5836) -> (x*y=w5835:dbl)
                          }
                        }
                        n3198 = case shown="True" w5794 {
                          tunnel: w5799 -> [w5824 w5829]
                          tunnel: w5800 -> [_ w5827]
                          tunnel: [w5824 w5828] -> w5797
                          tunnel: w5798 -> [w5823 w5826]
                          tunnel: [w5823 w5825] -> w5796
                          frame False {
                          }
                          frame True {
                            n3199 = Multiply(x=w5827, y=w5826) -> (x*y=w5825:dbl)
                            n3200 = Multiply(x=w5827, y=w5829) -> (x*y=w5828:dbl)
                          }
                        }
                        n3201 = local read "SIG LAB01-2"() -> (w5819:T2)
                        n3202 = local read "SIG LAB01-1"() -> (w5821:T2)
                        n3203 = Bundle By Name(cluster=w5821, "Tmp Live"=w5803, "Tmp Neut"=w5801) -> (w5820:T2)
                        n3204 = Bundle By Name(cluster=w5819, "Tmp Live"=w5797, "Tmp Neut"=w5796) -> (w5818:T2)
                        n3205 = local write "SIG LAB01-1"(w5820) -> ()
                        n3206 = local write "SIG LAB01-2"(w5818) -> ()
                      }
                      frame #2 {
                        n3207 = case shown="True" w5851 {
                          tunnel: [w5882 w5883] -> w5867
                          tunnel: w5850 -> [_ w5883]
                          frame False {
                            n3208 = local read "CAL LAB02"() -> (w5882:T15)
                          }
                          frame True {
                          }
                        }
                        n3209 = local read "LAB02 TEMP"() -> (w5858:T12)
                        n3210 = local read "TEMP LA02"() -> (w5857:T9)
                        n3211 = call "sub vi - temperature delay v4.vi"("2-run"=w5839, "1-run"=w5840, "temp values IN"=w5857, "temp signals"=w5858) -> ("T2-N"=w5852:dbl, "T2-L"=w5853:dbl, "T1-N"=w5854:dbl, "T1-L"=w5855:dbl, "temp values OUT"=w5856:T44)  [unwired: 3 in]
                        n3212 = Unbundle By Name(w5867) -> ("1 (TL) cal"=w5862:dbl, "1 (TN) cal"=w5861:dbl, "2 (TL) cal"=w5860:dbl, "2 (TN) cal"=w5859:dbl)  [unwired: 6 out]
                        n3213 = local write "TEMP LA02"(w5856) -> ()
                        n3214 = Multiply(x=w5855, y=w5862) -> (x*y=w5848:dbl)
                        n3215 = Multiply(x=w5854, y=w5861) -> (x*y=w5847:dbl)
                        n3216 = Multiply(x=w5853, y=w5860) -> (x*y=w5844:dbl)
                        n3217 = Multiply(x=w5852, y=w5859) -> (x*y=w5843:dbl)
                        n3218 = case shown="True" w5840 {
                          tunnel: w5848 -> [w5876 w5881]
                          tunnel: w5849 -> [_ w5879]
                          tunnel: [w5876 w5880] -> w5846
                          tunnel: w5847 -> [w5875 w5878]
                          tunnel: [w5875 w5877] -> w5845
                          frame False {
                          }
                          frame True {
                            n3219 = Multiply(x=w5879, y=w5878) -> (x*y=w5877:dbl)
                            n3220 = Multiply(x=w5879, y=w5881) -> (x*y=w5880:dbl)
                          }
                        }
                        n3221 = case shown="True" w5839 {
                          tunnel: w5844 -> [w5869 w5874]
                          tunnel: w5849 -> [_ w5872]
                          tunnel: [w5869 w5873] -> w5842
                          tunnel: w5843 -> [w5868 w5871]
                          tunnel: [w5868 w5870] -> w5841
                          frame False {
                          }
                          frame True {
                            n3222 = Multiply(x=w5872, y=w5871) -> (x*y=w5870:dbl)
                            n3223 = Multiply(x=w5872, y=w5874) -> (x*y=w5873:dbl)
                          }
                        }
                        n3224 = local read "SIG LAB02-2"() -> (w5864:T2)
                        n3225 = local read "SIG LAB02-1"() -> (w5866:T2)
                        n3226 = Bundle By Name(cluster=w5866, "Tmp Live"=w5846, "Tmp Neut"=w5845) -> (w5865:T2)
                        n3227 = Bundle By Name(cluster=w5864, "Tmp Live"=w5842, "Tmp Neut"=w5841) -> (w5863:T2)
                        n3228 = local write "SIG LAB02-1"(w5865) -> ()
                        n3229 = local write "SIG LAB02-2"(w5863) -> ()
                      }
                      frame #3 {
                        n3230 = case shown="False" w5896 {
                          tunnel: [w5927 w5928] -> w5912
                          tunnel: w5895 -> [_ w5928]
                          frame False {
                            n3231 = local read "CAL LAB03"() -> (w5927:T14)
                          }
                          frame True {
                          }
                        }
                        n3232 = local read "TEMP LA03"() -> (w5902:T9)
